vi "Write Solenoids.vi"(8 "error in (no error)":errorcluster, 10 "Solenoids":T1, 11 "Pneumatics in":refnum<class "Pneumatics.lvclass">) -> (0 "error out":errorcluster, 3 "Pneumatics out":refnum<class "Pneumatics.lvclass">)   [LabVIEW 2018, in "Pneumatics control.lvlib" / "Pneumatics.lvclass"]
uses:
  Pneumatics.lvclass
  TypeDefs/Solenoids.ctl
  Solenoids/Solenoids.lvclass
  Pneumatics.lvclass/Pneumatics.ctl
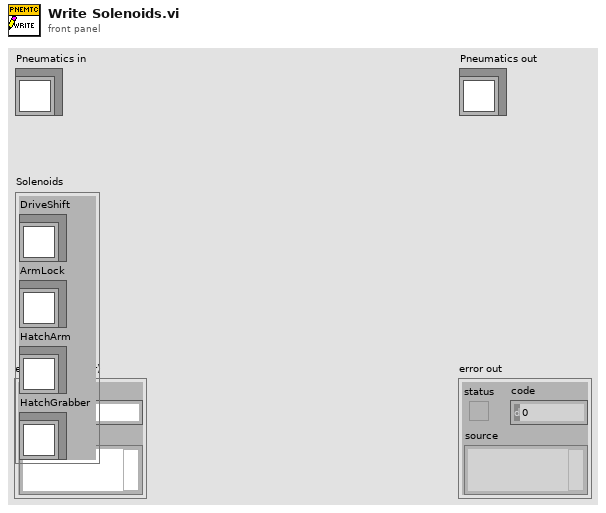
[diagram p1: front panel]
types:
  T1 = typedef "Pneumatics control.lvlib/Pneumatics.lvclass/Solenoids.ctl" = cluster{"DriveShift":refnum<class "Solenoids.lvclass">, "ArmLock":refnum<class "Solenoids.lvclass">, "HatchArm":refnum<class "Solenoids.lvclass">, "HatchGrabber":refnum<class "Solenoids.lvclass">}
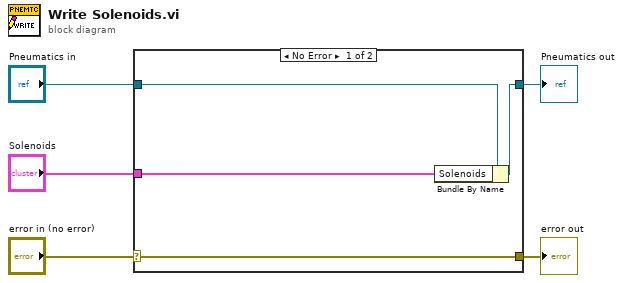
[diagram p0: block diagram]
diagram:
  n1 = case shown="No Error" "error in (no error)" {
    selector: "error in (no error)" -> [w9 w10]
    tunnel: [w9 w10] -> w4
    tunnel: [w7 w11] -> w2
    tunnel: "Pneumatics in" -> [w8 w11]
    tunnel: "Solenoids" -> [w6 _]
    frame No Error {
      n2 = Bundle By Name(cluster=w8, "Solenoids"=w6) -> (w7:refnum<class "Pneumatics.lvclass">)
    }
    frame Error {
    }
  }
  "error out" <- w4
  "Pneumatics out" <- w2
